vi "Correct Aim.vi"(8 "error in":errorcluster, 11 "Image In":T1) -> (0 "error out":errorcluster, 3 "Image Out":T1)   [LabVIEW 2012]
uses:
  <vilib>/vision/Image Controls.llb/IMAQ Image.ctl
  Rec Targeting.vi
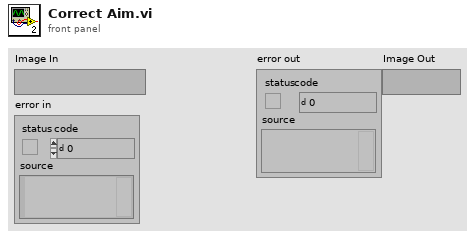
[diagram p1: front panel]
types:
  T1 = typedef "IMAQ Image.ctl" = refnum<image>
  T2 = typedef "WPI_CameraDevRef.ctl" = cluster{"Camera Address":string, "CameraStatus":errorcluster, "Acquire Image Notifier":refnum<notifier>}
  T3 = typedef "WPI_CameraImageSize.ctl" = enum16{"640x480", "320x240", "160x120"}
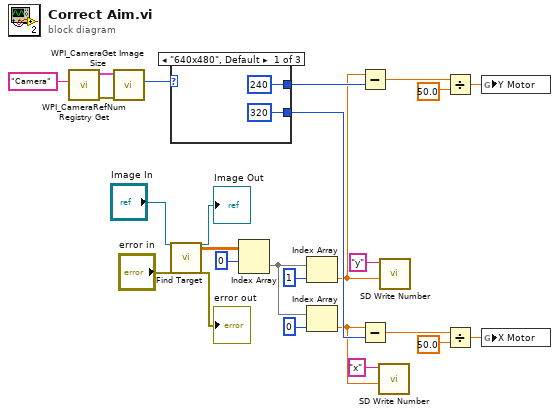
[diagram p0: block diagram]
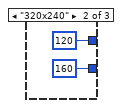
[diagram p2: hidden frame]
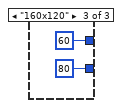
[diagram p3: hidden frame]
diagram:
  n1 = call <vilib>:"WPI_CameraRefNum Registry Get.vi"("refnum name"="Camera") -> ("error out"=w10:errorcluster, "CameraDevRef"=w9:T2)  [unwired: 9 in]
  n2 = call <vilib>:"WPI_CameraGet Image Size.vi"("error in (no error)"=w10, "CameraDevRef"=w9) -> ("Image Size"=w7:T3)  [unwired: 7 in, 2 out]
  n3 = case shown="\"640x480\", Default" w7 {
    tunnel: [320 160 80] -> w6
    tunnel: [240 120 60] -> w5
    frame "640x480", Default {
    }
    frame "320x240" {
    }
    frame "160x120" {
    }
  }
  n4 = call "Find Target.vi"("Image In"="Image In", "error in"="error in") -> ("Image Out"=→"Image Out":T1, "Particle Measurements (Pixels) (Particle Analysis 1)"=w25:dbl[][], "error out"=→"error out":errorcluster)  [unwired: 23 in]
  n5 = Index Array(array=w25, index (row)=0) -> (element=w21:dbl[])  [unwired: 1 in]
  n6 = Index Array(array=w21, index=1) -> (element=w1:dbl)
  n7 = Index Array(array=w21, index=0) -> (element=w2:dbl)
  n8 = Subtract(x=w1, y=w5) -> (x-y=w18:dbl)
  n9 = Subtract(x=w2, y=w6) -> (x-y=w16:dbl)
  n10 = call <vilib>:"SD Write Number.vi"("Numeric"=w2, "Name"="x") -> ()  [unwired: 8 in, 2 out]
  n11 = call <vilib>:"SD Write Number.vi"("Numeric"=w1, "Name"="y") -> ()  [unwired: 8 in, 2 out]
  n12 = Divide(x=w18, y=50.0) -> (x/y=w13:dbl)
  n13 = Divide(x=w16, y=50.0) -> (x/y=w14:dbl)
  n14 = global write "Rec Targeting.vi" "Y Motor"(w13) -> ()
  n15 = global write "Rec Targeting.vi" "X Motor"(w14) -> ()
